vi "Malab Style Vector.vi"(9 "dt":dbl, 10 "b":dbl, 11 "a":dbl) -> (3 "Vector":dbl[](array[numeric]))   [LabVIEW 2011]
doc: "An implementation of the Matlab command \"a:dt:b\"."
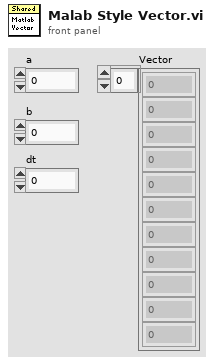
[diagram p1: front panel]
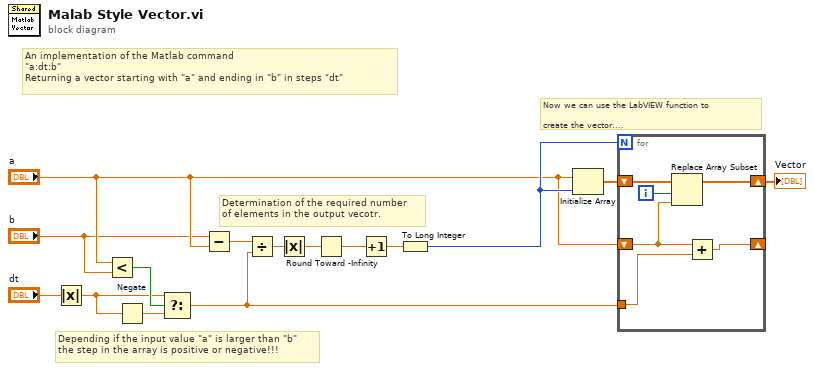
[diagram p0: block diagram]
diagram:
  # "Now we can use the LabVIEW function to\n\ncreate the vector...."
  # "Determination of the required number\nof elements in the output vecotr."
  # "Depending if the input value \"a\" is larger than \"b\"\nthe step in the array is positive or negative!!!"
  # "An implementation of the Matlab command\n\"a:dt:b\"\nReturning a vector starting with \"a\" and ending in \"b\" in steps \"dt\""
  n1 = Absolute Value(x="dt") -> (abs(x)=w2:dbl)
  n2 = Less?(x="a", y="b") -> (x < y?=w4:bool)
  n3 = Negate(x=w2) -> (-x=w3:dbl)
  n4 = Select(t=w2, s=w4, f=w3) -> (s? t:f=w1:dbl)
  n5 = Subtract(x="b", y="a") -> (x-y=w15:dbl)
  n6 = Divide(x=w15, y=w1) -> (x/y=w14:dbl)
  n7 = Absolute Value(x=w14) -> (abs(x)=w13:dbl)
  n8 = Round Toward -Infinity(1:w13) -> (0:w12:dbl)
  n9 = Increment(x=w12) -> (x+1=w11:dbl)
  n10 = To Long Integer(number=w11) -> (32bit integer=w9:i32)
  n11 = Initialize Array("a", w9) -> (w10:dbl[])
  n12 = for {
    N: w9 -> [_]
    shift-right: [w17] -> _
    shift-left: "a" -> [w19]
    tunnel: w1 -> [w18]
    shift-right: [w16] -> w8
    shift-left: w10 -> [w21]
    i -> [w20]
    n13 = Replace Array Subset(array=w21, new element=w19, index=w20) -> (w16:dbl[])
    n14 = Add(x=w19, y=w18) -> (x+y=w17:dbl)
  }
  "Vector" <- w8
